vi "Add To Storage.vi"(8 "error in":errorcluster, 9 "Item Name":string, 10 "Item node":refnum<k20>, 11 "Item Ref in":refnum<data-value>) -> (0 "error out":errorcluster, 3 "Item Ref out":refnum<data-value>)   [LabVIEW 2024, in "Config File Parser.lvlib"]
uses:
  Config File Parser.lvlib
  Item/Item.lvclass
  Custom Device Config/Custom Device Config.lvclass
  <vilib>/xml/Close Reference(Node).vi
  Property/Property.lvclass
  Channel/Channel.lvclass
  Section/Section.lvclass
  <vilib>/xml/NI_XML.lvlib
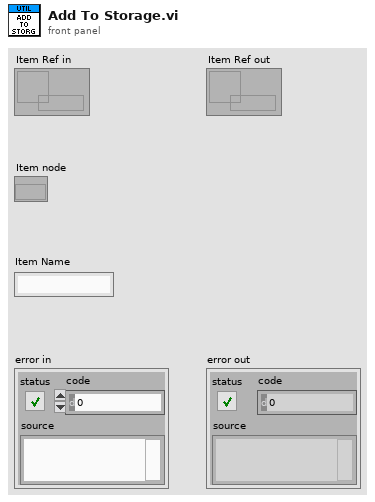
[diagram p1: front panel]
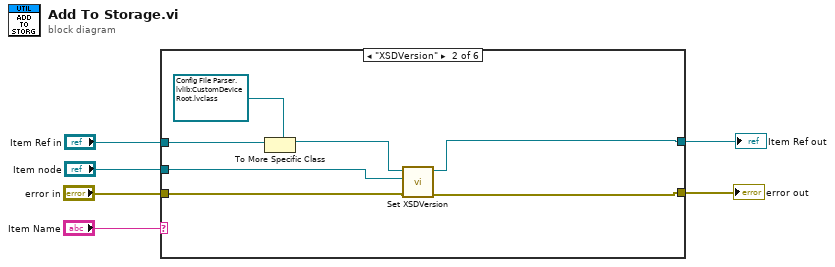
[diagram p0: block diagram]
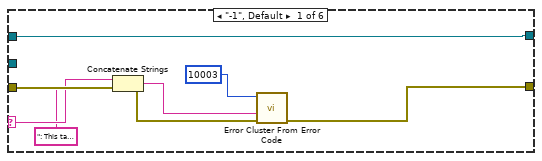
[diagram p2: hidden frame]
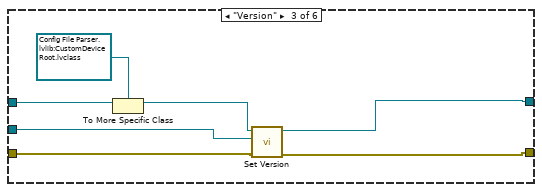
[diagram p3: hidden frame]
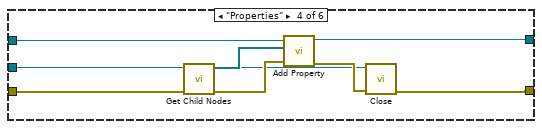
[diagram p4: hidden frame]
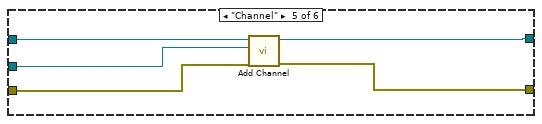
[diagram p5: hidden frame]
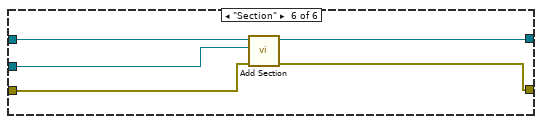
[diagram p6: hidden frame]
diagram:
  n1 = case shown="\"XSDVersion\"" "Item Name" {
    selector: "Item Name" -> [w10 _ _ _ _ _]
    tunnel: "Item node" -> [_ w18 w25 w30 w38 w43]
    tunnel: "error in" -> [w13 w20 w27 w35 w40 w45]
    tunnel: [w12 w19 w26 w33 w39 w44] -> w5
    tunnel: [w7 w17 w23 w29 w37 w42] -> w1
    tunnel: "Item Ref in" -> [w7 w16 w24 w28 w36 w41]
    frame "-1", Default {
      n2 = Concatenate Strings(w10, ": This tag is not allowed. " ("string")) -> (w9:string)
      n3 = call <vilib>:"Error Cluster From Error Code.vi"("error in (no error)"=w13, "error message (\"\")"=w9, "error code (0)"=10003 ("Code")) -> ("error out"=w12:errorcluster)  [unwired: 6 in]
    }
    frame "XSDVersion" {
      n4 = To More Specific Class(target class=refnum<data-value> refnum ("Custom Device Config Ref"), reference=w16) -> (specific class reference=w14:refnum<data-value>)  [unwired: 1 in, 1 out]
      n5 = call "Set XSDVersion.vi"("error in"=w20, "XML Node"=w18, "Custom Device Config Ref in"=w14) -> ("error out"=w19:errorcluster, "Custom Device Config Ref out"=w17:refnum<data-value>)  [unwired: 7 in]
    }
    frame "Version" {
      n6 = To More Specific Class(target class=refnum<data-value> refnum ("Custom Device Config Ref"), reference=w24) -> (specific class reference=w21:refnum<data-value>)  [unwired: 1 in, 1 out]
      n7 = call "Set Version.vi"("error in"=w27, "XML Node"=w25, "Custom Device Config Ref in"=w21) -> ("error out"=w26:errorcluster, "Custom Device Config Ref out"=w23:refnum<data-value>)  [unwired: 7 in]
    }
    frame "Properties" {
      n8 = call "Get Child Nodes.vi"("error in"=w35, "Node"=w30) -> ("error out"=w34:errorcluster, "Child Nodes"=w31:refnum<k20>[])  [unwired: 8 in]
      n9 = call "Add Property.vi"("error in"=w34, "Property Nodes"=w31, "Item Ref in"=w28) -> ("error out"=w32:errorcluster, "Item Ref out"=w29:refnum<data-value>)  [unwired: 7 in]
      n10 = call-poly <vilib>:"Close.vi"("error in (no error)"=w32, "node"=w30) -> ("error out"=w33:errorcluster)  [unwired: 7 in]
    }
    frame "Channel" {
      n11 = call "Add Channel.vi"("error in"=w40, "Channel Node"=w38, "Item Ref in"=w36) -> ("error out"=w39:errorcluster, "Item Ref out"=w37:refnum<data-value>)  [unwired: 7 in]
    }
    frame "Section" {
      n12 = call "Add Section.vi"("error in"=w45, "Section Node"=w43, "Item Ref in"=w41) -> ("error out"=w44:errorcluster, "Item Ref out"=w42:refnum<data-value>)  [unwired: 7 in]
    }
  }
  "error out" <- w5
  "Item Ref out" <- w1
